vi "Constants.vi"() -> ()   [LabVIEW 2019, in "Listener.lvclass"]
uses:
  Listener.lvclass
panel:
  in  "AK TCP Data Length":dbl=12.0
  in  "Current Command Code":string="Code"
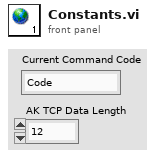
[diagram p1: front panel]
diagram:
